vi "判断是否构成三角形.vi"(0 "B":dbl, 1 "C":dbl, 4 "A":dbl) -> (6 "A、B、C是否构成三角形":bool)   [LabVIEW 2018]
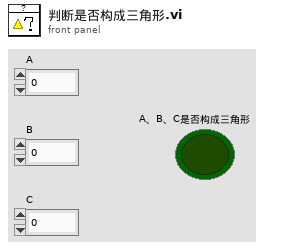
[diagram p1: front panel]
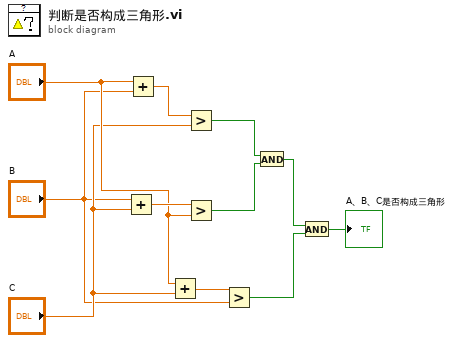
[diagram p0: block diagram]
diagram:
  n1 = Add(x="B", y="C") -> (x+y=w10:dbl)
  n2 = Add(x="A", y="B") -> (x+y=w11:dbl)
  n3 = Add(x="A", y="C") -> (x+y=w7:dbl)
  n4 = Greater?(x=w11, y="C") -> (0:w5:bool)
  n5 = Greater?(x=w10, y="A") -> (0:w4:bool)
  n6 = Greater?(x=w7, y="B") -> (0:w2:bool)
  n7 = And(x=w5, y=w4) -> (x .and. y?=w3:bool)
  n8 = And(x=w3, y=w2) -> (x .and. y?=→"A、B、C是否构成三角形":bool)
